vi "Set Channel N.vi"(0 "EPU452 in":refnum<class "EPU452.lvclass">, 5 "Channel":T1, 7 "Function":string, 9 "Argument/s":string, 11 "error in (no error)":errorcluster) -> (4 "EPU452 out":refnum<class "EPU452.lvclass">, 8 "Response":string, 15 "error out":errorcluster)   [LabVIEW 2018, in "EPU452.lvclass"]
uses:
  EPU452.lvclass
  Controls/Channels.ctl
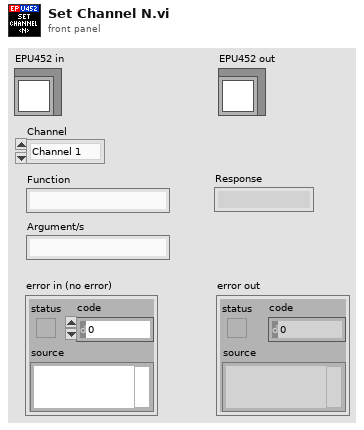
[diagram p1: front panel]
types:
  T1 = typedef "EPU452.lvclass/Channels.ctl" = enum16{"Channel 1", "Channel 2", "Channel 3", "Channel 4"}
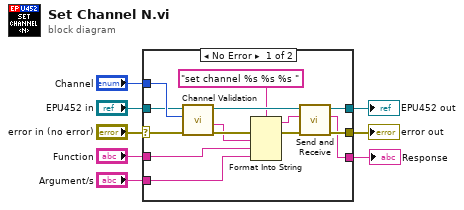
[diagram p0: block diagram]
diagram:
  n1 = case shown="No Error" "error in (no error)" {
    selector: "error in (no error)" -> [w20 w24]
    tunnel: [w10 w24] -> w7
    tunnel: [w11 w23] -> w5
    tunnel: "EPU452 in" -> [w21 w23]
    tunnel: "Channel" -> [w22 _]
    tunnel: "Function" -> [w17 _]
    tunnel: "Argument/s" -> [w16 _]
    tunnel: [w9 _] -> w1
    frame No Error {
      n2 = call "Channel Validation.vi"("error in (no error)"=w20, "Channel in"=w22, "EPU452 in"=w21) -> ("error out"=w19:errorcluster, "Channel"=w18:string, "EPU452 out"=w14:refnum<class "EPU452.lvclass">)  [unwired: 5 in, 1 out]
      n3 = Format Into String(format string="set channel %s %s %s ", error in=w19, w18, w17, w16) -> (resulting string=w12:string, error out=w15:errorcluster)  [unwired: 1 in]
      n4 = call "Send and Receive.vi"("error in (no error)"=w15, "Command"=w12, "EPU452 in"=w14) -> ("error out"=w10:errorcluster, "Response"=w9:string, "EPU452 out"=w11:refnum<class "EPU452.lvclass">)  [unwired: 6 in]
    }
    frame Error {
    }
  }
  "error out" <- w7
  "EPU452 out" <- w5
  "Response" <- w1
